vi "Change Setting.vi"(8 "error in (no error)":errorcluster, 10 "Change setting mode":T1, 11 "Toggle 6 in":refnum<class "Toggle 6.lvclass">) -> (0 "error out":errorcluster, 1 "Changes":cluster{"Name":string, "Value":string}[](array[cluster]), 2 "Last setting":bool, 3 "Toggle 6 out":refnum<class "Toggle 6.lvclass">)   [LabVIEW 2020, in "Toggle 6.lvclass"]
uses:
  Toggle 6.lvclass
  C:/Sandbox/Git_Sandbox/WiSpry Test Framework source code (LV20)/WiSpry Test Framework/Devices/Device.lvclass
  Controls/Change setting mode enum.ctl
  Instruments/Power Supply/Power Supply.lvclass
  Device.lvclass
  PIC-device/PIC-Device.lvclass
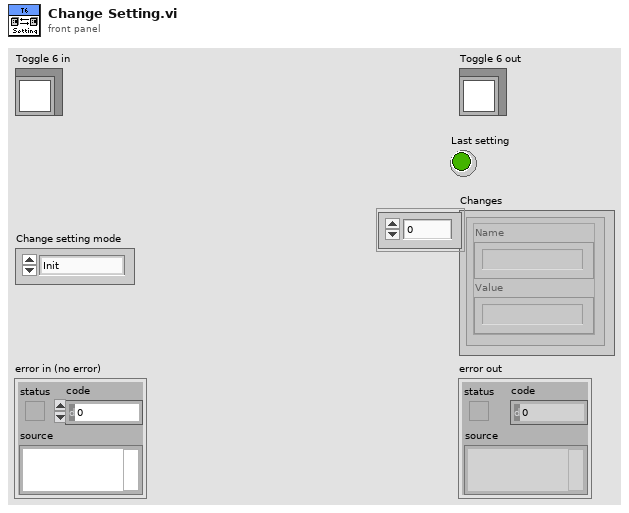
[diagram p1: front panel]
types:
  T1 = typedef "PIC-Device.lvclass/Change setting mode enum.ctl" = enum16{"Init", "Next", "Reset"}
  T2 = typedef "Toggle 6.lvclass/Test Sequence.ctl" = cluster{"Charge Pump Settings":T3[], "Charge Pump Values":dbl[], "Efuse Register Array":T3[], "Efuse Array":T4[], "Cap Register Array":T3[], "Cap Value Array":cluster{"Register Number":u32, "Value":dbl}[]}
  T3 = typedef "PIC-Device.lvclass/Register to Write.ctl" = cluster{"Register":u32, "Value":u32, "Dev Address":u32, "Physical Adress":u32}
  T4 = typedef "Toggle 6.lvclass/EFuse modes enum.ctl" = enum16{"On", "Off", "Both On and Off"}
  T5 = typedef "Device.lvclass/DC Offset Cluster.ctl" = cluster{"Enable":bool, "Use Array":bool, "Array":dbl[], "To From Cluster":cluster{"From":dbl, "To":dbl, "Step":dbl}, "Current Value":dbl, "DC Offset":refnum<class "Power Supply.lvclass">}
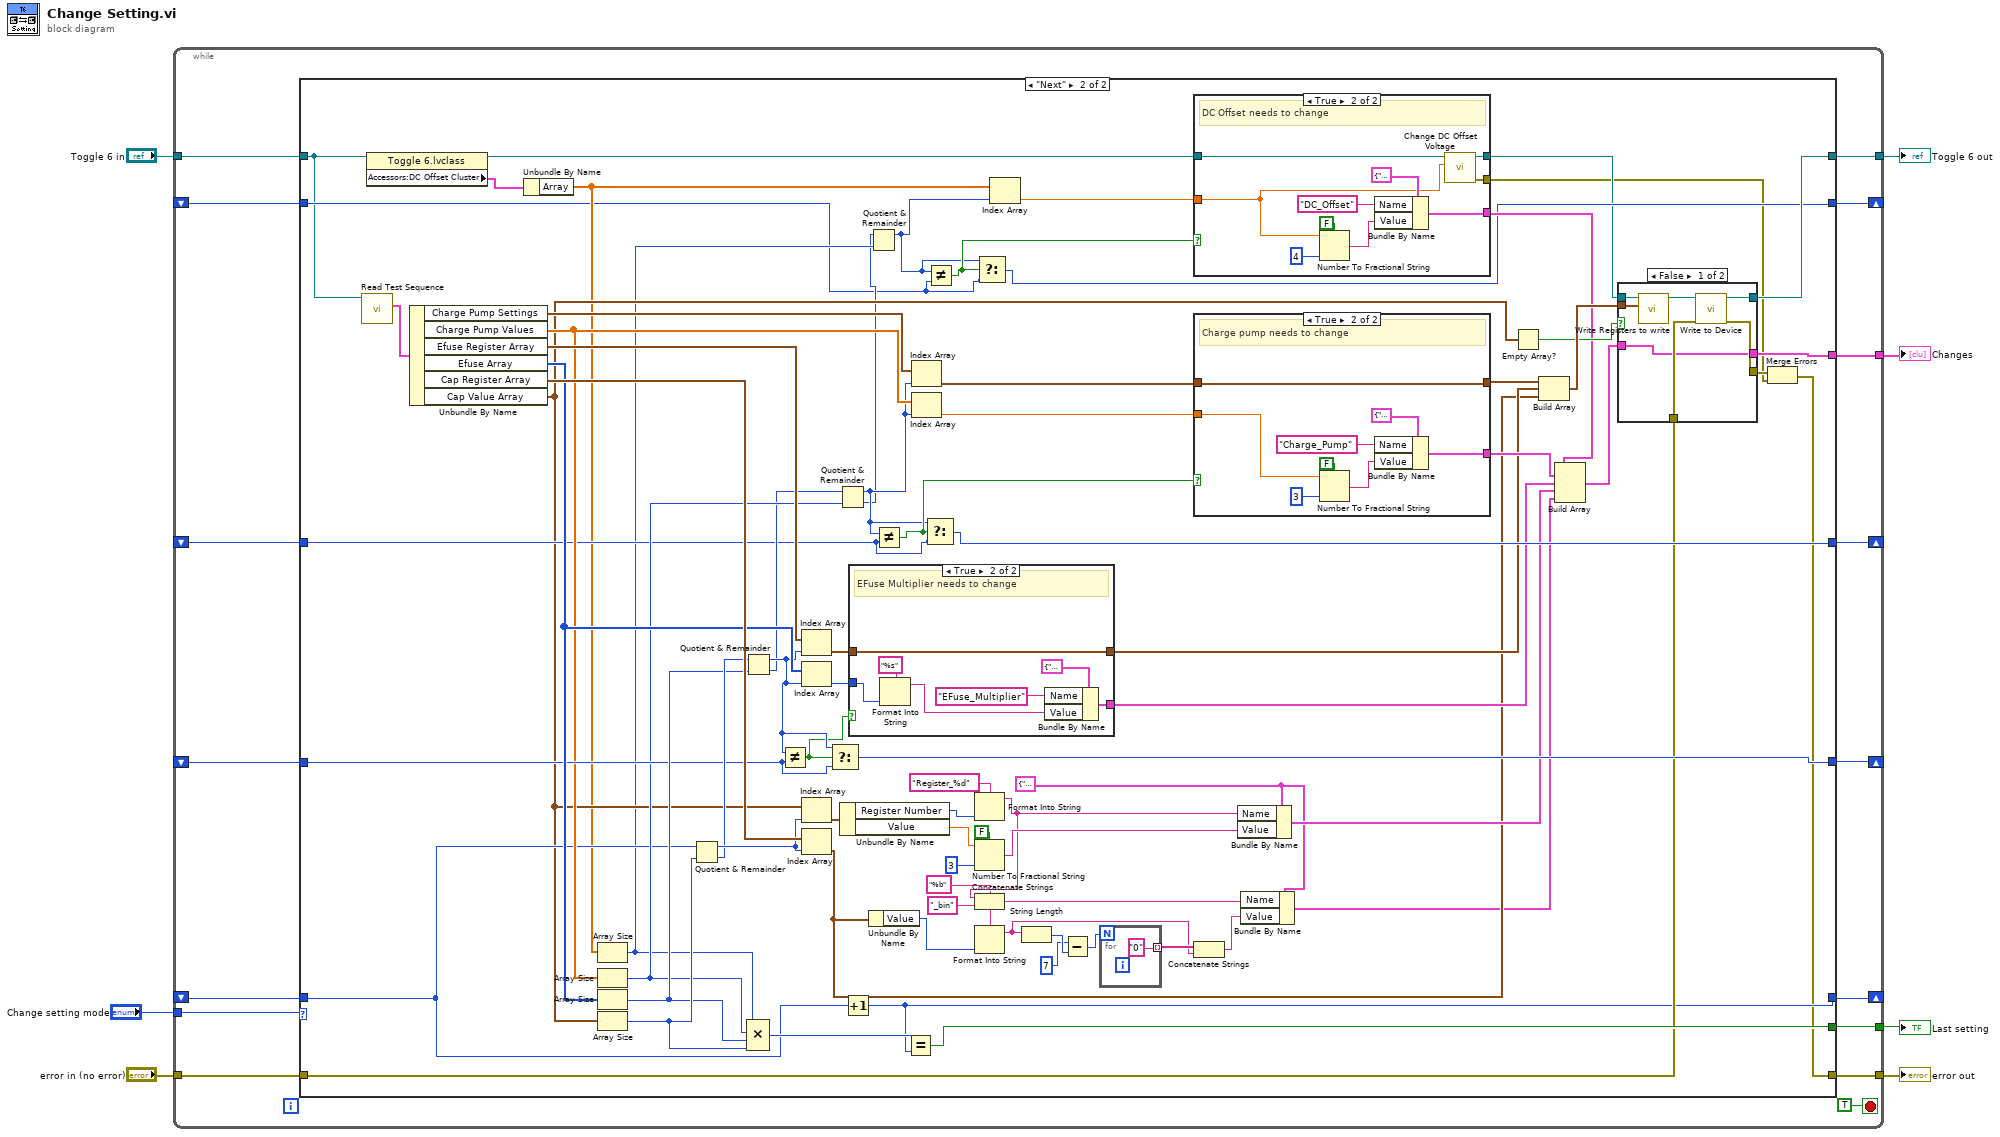
[diagram p0: block diagram]
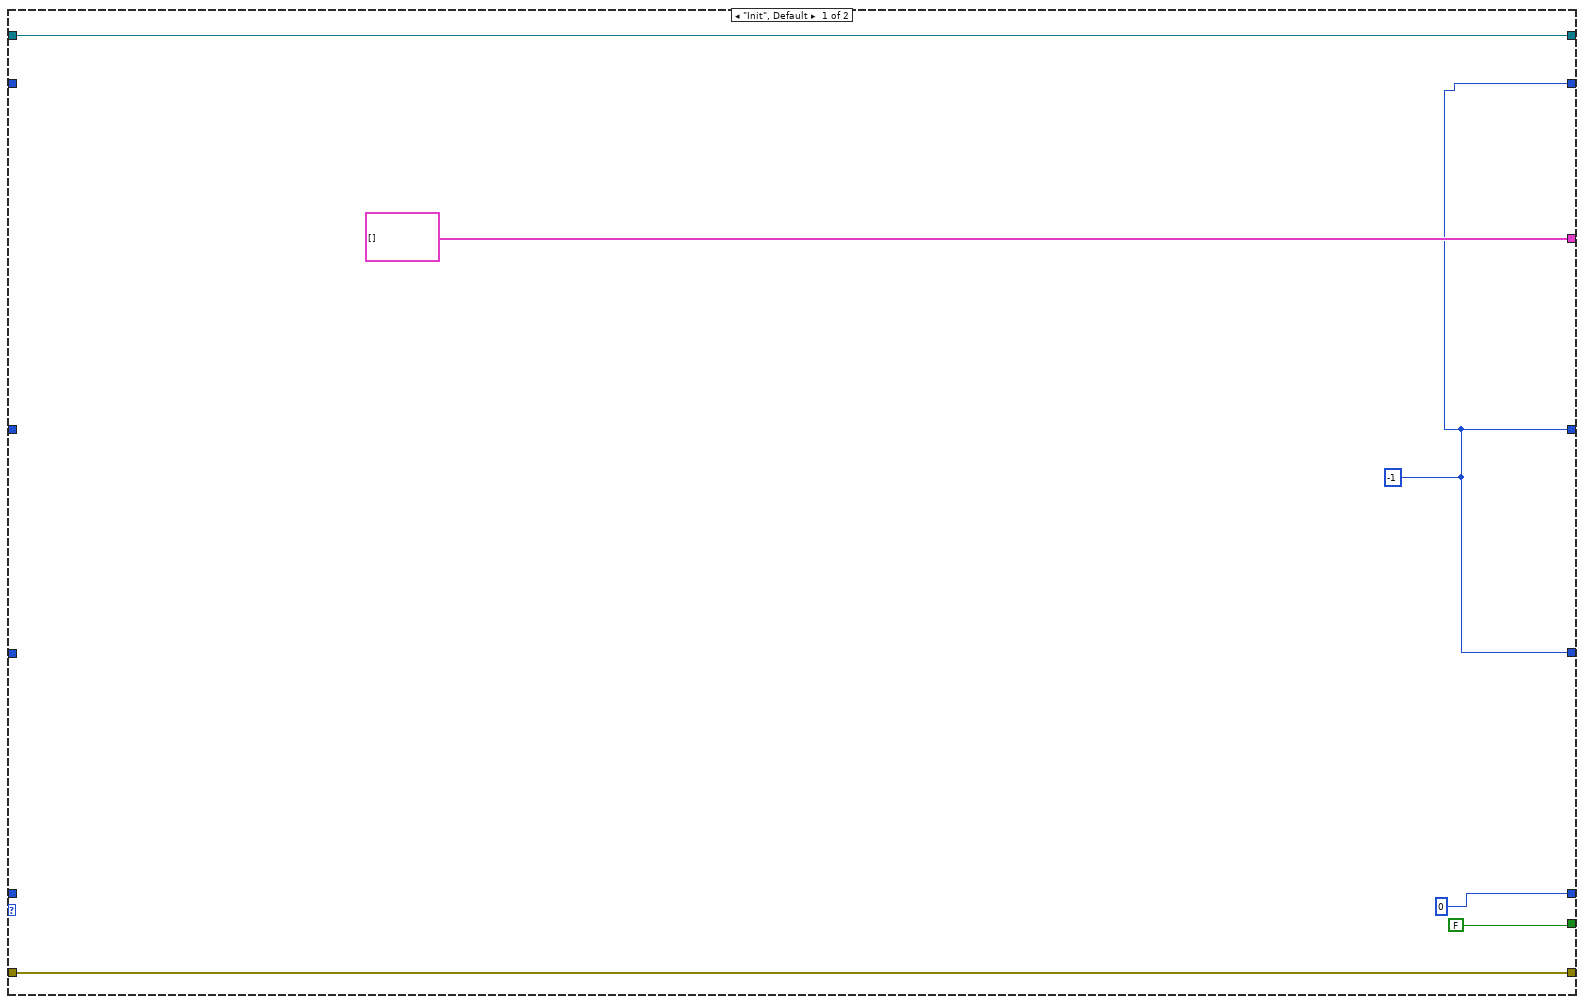
[diagram p2: hidden frame]
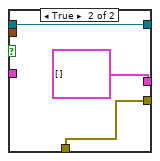
[diagram p4: hidden frame]
diagram:
  n1 = while {
    tunnel: "error in (no error)" -> [w21]
    tunnel: "Change setting mode" -> [w22]
    tunnel: "Toggle 6 in" -> [w17]
    tunnel: [w20] -> w4
    shift-right: [w19] -> _
    shift-left: _ -> [w18]
    tunnel: [w16] -> w3
    tunnel: [w15] -> w2
    shift-right: [w14] -> _
    shift-left: _ -> [w12]
    shift-right: [w13] -> _
    shift-left: _ -> [w11]
    tunnel: [w10] -> w1
    shift-right: [w9] -> _
    shift-left: _ -> [w8]
    stop <- TRUE stop-if-true
    n2 = case shown="\"Next\"" w22 {
      tunnel: w21 -> [w25 w68]
      tunnel: [FALSE w104] -> w20
      tunnel: [0 w45] -> w19
      tunnel: w18 -> [_ w50]
      tunnel: w17 -> [w26 w31]
      tunnel: [cluster{"Name":string, "Value":string}[] [] ("Changes") w47] -> w16
      tunnel: [w26 w69] -> w15
      tunnel: [w24 w88] -> w14
      tunnel: [w24 w79] -> w13
      tunnel: w12 -> [_ w89]
      tunnel: w11 -> [_ w80]
      tunnel: [w25 w36] -> w10
      tunnel: [w24 w39] -> w9
      tunnel: w8 -> [_ w34]
      frame "Init", Default {
        w24 = -1
      }
      frame "Next" {
        w63 = cluster{"Name":string, "Value":string} {"Name"="", "Value"=""} ("Change")
        n3 = call-dynamic "Read Test Sequence.vi"("Toggle 6 in"=w31) -> ("Test Sequence"=w106:T2)  [unwired: 9 in, 1 out]
        n4 = property class="Toggle 6.lvclass"(reference=w31) -> (reference out=w30:refnum<class "Toggle 6.lvclass">, "Accessors:DC Offset Cluster"=w32:T5)  [unwired: 1 in, 1 out]
        n5 = Unbundle By Name(w106) -> ("Charge Pump Settings"=w82:T3[], "Charge Pump Values"=w81:dbl[], "Efuse Register Array"=w92:T3[], "Efuse Array"=w91:T4[], "Cap Register Array"=w102:T3[], "Cap Value Array"=w49:cluster{"Register Number":u32, "Value":dbl}[])
        n6 = Unbundle By Name(w32) -> ("Array"=w42:dbl[])
        n7 = Array Size(array=w42) -> (size(s)=w41:i32)
        n8 = Array Size(array=w81) -> (size(s)=w84:i32)
        n9 = Array Size(array=w91) -> (size(s)=w93:i32)
        n10 = Array Size(array=w49) -> (size(s)=w103:i32)
        n11 = Quotient & Remainder(x=w50, y=w103) -> (x-y*floor(x/y)=w101:i32, floor(x/y)=w94:i32)
        n12 = Quotient & Remainder(x=w94, y=w93) -> (x-y*floor(x/y)=w90:i32, floor(x/y)=w83:i32)
        n13 = Compound Arithmetic op=MULTIPLY(w41, w84, w93, w103) -> (w105:i32)
        n14 = Not Equal?(x=w90, y=w89) -> (x != y?=w87:bool)
        n15 = Index Array(array=w92, index=w90) -> (element=w86:T3)
        n16 = Index Array(array=w91, index=w90) -> (element=w85:T4)
        n17 = Index Array(array=w49, index=w101) -> (element=w100:cluster{"Register Number":u32, "Value":dbl})
        n18 = Index Array(array=w102, index=w101) -> (element=w62:T3)
        n19 = Select(t=w90, s=w87, f=w89) -> (s? t:f=w88:i32)
        n20 = Quotient & Remainder(x=w83, y=w84) -> (x-y*floor(x/y)=w66:i32, floor(x/y)=w40:i32)
        n21 = Unbundle By Name(w100) -> ("Register Number"=w99:u32, "Value"=w96:dbl)
        n22 = Increment(x=w50) -> (x+1=w45:i32)
        n23 = case shown="True" w87 {
          tunnel: w86 -> [_ w137]
          tunnel: w85 -> [_ w142]
          tunnel: [_ w138] -> w74
          tunnel: [_ w137] -> w71
          frame False {
          }
          frame True {
            # "EFuse Multiplier needs to change"
            n24 = Format Into String(format string="%s", w142) -> (resulting string=w139:string)  [unwired: 2 in, 1 out]
            n25 = Bundle By Name(cluster=cluster{"Name":string, "Value":string} {"Name"="", "Value"=""} ("Change"), "Name"="EFuse_Multiplier", "Value"=w139) -> (w138:cluster{"Name":string, "Value":string})
          }
        }
        n26 = Unbundle By Name(w62) -> ("Value"=w60:u32)
        n27 = Quotient & Remainder(x=w40, y=w41) -> (x-y*floor(x/y)=w33:i32)  [unwired: 1 out]
        n28 = Not Equal?(x=w66, y=w80) -> (x != y?=w78:bool)
        n29 = Equal?(x=w105, y=w45) -> (x = y?=w104:bool)
        n30 = Index Array(array=w82, index=w66) -> (element=w77:T3)
        n31 = Index Array(array=w81, index=w66) -> (element=w76:dbl)
        n32 = Select(t=w66, s=w78, f=w80) -> (s? t:f=w79:i32)
        n33 = Not Equal?(x=w33, y=w34) -> (x != y?=w38:bool)
        n34 = Format Into String(format string="Register_%d", w99) -> (resulting string=w65:string)  [unwired: 2 in, 1 out]
        n35 = Number To Fractional String(use system decimal point (T)=FALSE, number=w96, precision (6)=i16 3) -> (F-format string=w97:string)  [unwired: 1 in]
        n36 = Concatenate Strings(w65, "_bin" ("string")) -> (w61:string)
        n37 = Format Into String(format string="%b", w60) -> (resulting string=w53:string)  [unwired: 2 in, 1 out]
        n38 = Select(t=w33, s=w38, f=w34) -> (s? t:f=w39:i32)
        n39 = Index Array(array=w42, index=w33) -> (element=w44:dbl)
        n40 = String Length(string=w53) -> (length=w57:i32)
        n41 = Subtract(x=7, y=w57) -> (x-y=w55:i32)
        n42 = for {
          N: w55 -> [_]
          tunnel: ["0"] -> w54 mode=indexing
        }
        n43 = case shown="True" w38 {
          tunnel: w44 -> [_ w108]
          tunnel: [_ w113] -> w43
          tunnel: w30 -> [w107 w111]
          tunnel: [w107 w110] -> w37
          tunnel: [_ w109] -> w35
          frame False {
          }
          frame True {
            # "DC Offset needs to change"
            n44 = Number To Fractional String(use system decimal point (T)=FALSE, number=w108, precision (6)=i16 4) -> (F-format string=w115:string)  [unwired: 1 in]
            n45 = Bundle By Name(cluster=cluster{"Name":string, "Value":string} {"Name"="", "Value"=""} ("Change"), "Name"="DC_Offset", "Value"=w115) -> (w113:cluster{"Name":string, "Value":string})
            n46 = call "Change DC Offset Voltage.vi"("DC Offset"=w108, "Device in"=w111) -> ("error out"=w109:errorcluster, "Device out"=w110:refnum<class "Toggle 6.lvclass">)  [unwired: 8 in]
          }
        }
        n47 = case shown="True" w78 {
          tunnel: w77 -> [_ w131]
          tunnel: w76 -> [_ w132]
          tunnel: [_ w131] -> w72
          tunnel: [_ w130] -> w75
          frame False {
          }
          frame True {
            # "Charge pump needs to change"
            n48 = Number To Fractional String(use system decimal point (T)=FALSE, number=w132, precision (6)=i16 3) -> (F-format string=w134:string)  [unwired: 1 in]
            n49 = Bundle By Name(cluster=cluster{"Name":string, "Value":string} {"Name"="", "Value"=""} ("Change"), "Name"="Charge_Pump", "Value"=w134) -> (w130:cluster{"Name":string, "Value":string})
          }
        }
        n50 = Concatenate Strings(w54, w53) -> (w52:string)
        n51 = Bundle By Name(cluster=w63, "Name"=w65, "Value"=w97) -> (w73:cluster{"Name":string, "Value":string})
        n52 = Bundle By Name(cluster=w63, "Name"=w61, "Value"=w52) -> (w58:cluster{"Name":string, "Value":string})
        n53 = Empty Array?(array=w49) -> (empty?=w48:bool)
        n54 = Build Array(w72, w71, w62) -> (w70:T3[])
        n55 = Build Array(w43, w75, w74, w73, w58) -> (w46:cluster{"Name":string, "Value":string}[])
        n56 = case shown="False" w48 {
          tunnel: w37 -> [w124 w127]
          tunnel: w70 -> [w123 _]
          tunnel: [w121 w127] -> w69
          tunnel: w68 -> [w120 w126]
          tunnel: [w119 w126] -> w67
          tunnel: [w118 cluster{"Name":string, "Value":string}[] []] -> w47
          tunnel: w46 -> [w118 _]
          frame False {
            n57 = call-dynamic "Write Registers to write.vi"("Registers to write"=w123, "Device in"=w124) -> ("Device out"=w122:refnum<class "Toggle 6.lvclass">)  [unwired: 9 in]
            n58 = call-dynamic "Write to Device.vi"("error in (no error)"=w120, "Device in"=w122) -> ("error out"=w119:errorcluster, "Device out"=w121:refnum<class "Toggle 6.lvclass">)  [unwired: 7 in, 1 out]
          }
          frame True {
          }
        }
        n59 = Merge Errors(w67, w35) -> (w36:errorcluster)
      }
    }
  }
  "error out" <- w1
  "Toggle 6 out" <- w2
  "Changes" <- w3
  "Last setting" <- w4
